vi "OpenSF.vi"(1 "Port number\nactuators":u16, 2 "Port number\nsensors":u16) -> (0 "connection IDs":T1)   [LabVIEW 2010]
panel:
  out "Error out\nactuators":errorcluster
  out "Error out\nsensors":errorcluster
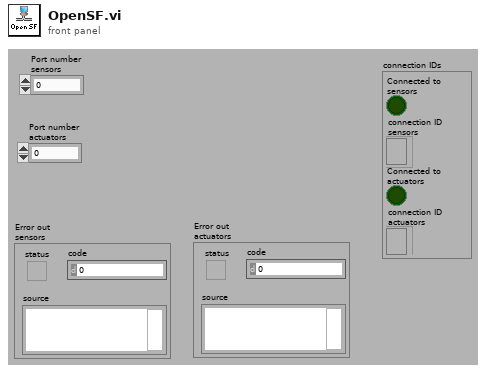
[diagram p1: front panel]
types:
  T1 = cluster{"Connected to\nsensors":bool, "connection ID\nsensors":refnum<k5>, "Connected to\nactuators":bool, "connection ID\nactuators":refnum<k5>}
  T2 = cluster{bool, "connection ID":refnum<k5>, bool, "connection ID":refnum<k5>}
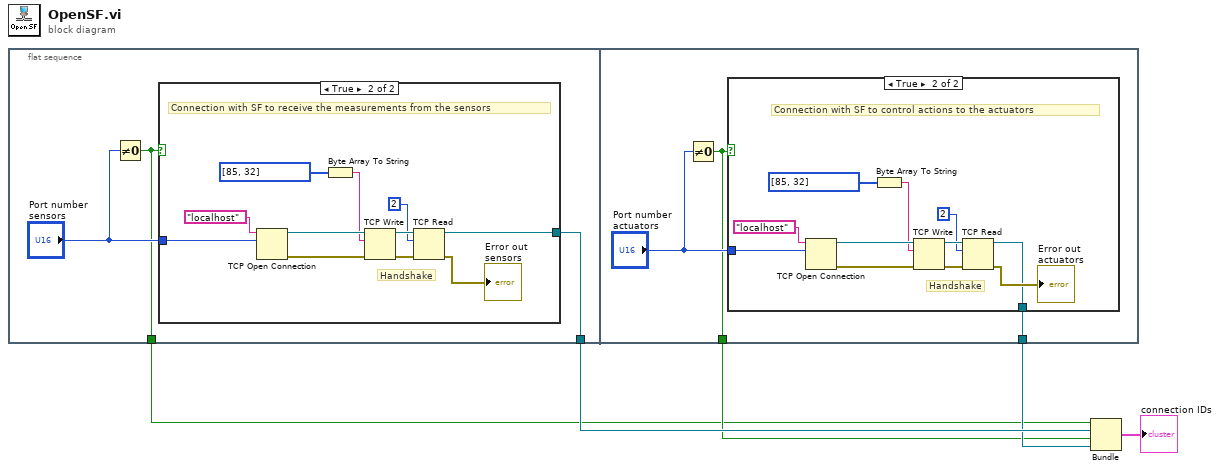
[diagram p0: block diagram]
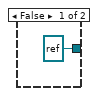
[diagram p2: hidden frame]
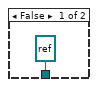
[diagram p3: hidden frame]
diagram:
  n1 = flat-sequence {
    tunnel: [w8] -> w5
    tunnel: [w6] -> w1
    tunnel: [w23] -> w4
    tunnel: [w21] -> w2
    frame #0 {
      n2 = Not Equal To 0?(x="Port number\nsensors") -> (x != 0?=w6:bool)
      n3 = case shown="True" w6 {
        tunnel: "Port number\nsensors" -> [_ w19]
        tunnel: [refnum<k5> refnum ("connection ID") w10] -> w8
        frame False {
        }
        frame True {
          # "Connection with SF to receive the measurements from the sensors"
          # "Handshake"
          n4 = TCP Open Connection(address="localhost", remote port or service name=w19) -> (connection ID=w16:refnum<k5>, error out=w15:errorcluster)  [unwired: 3 in]
          n5 = Byte Array To String(unsigned byte array=u8[] [85, 32]) -> (string=w12:string)
          n6 = TCP Write(connection ID=w16, data in=w12, error in (no error)=w15) -> (connection ID out=w17:refnum<k5>, error out=w18:errorcluster)  [unwired: 1 in, 1 out]
          n7 = TCP Read(connection ID=w17, bytes to read=2, error in (no error)=w18) -> (connection ID out=w10:refnum<k5>, error out=→"Error out\nsensors":errorcluster)  [unwired: 2 in, 1 out]
        }
      }
    }
    frame #1 {
      n8 = Not Equal To 0?(x="Port number\nactuators") -> (x != 0?=w21:bool)
      n9 = case shown="True" w21 {
        tunnel: "Port number\nactuators" -> [_ w34]
        tunnel: [refnum<k5> refnum ("connection ID") w25] -> w23
        frame False {
        }
        frame True {
          # "Connection with SF to control actions to the actuators"
          # "Handshake"
          n10 = TCP Open Connection(address="localhost", remote port or service name=w34) -> (connection ID=w31:refnum<k5>, error out=w30:errorcluster)  [unwired: 3 in]
          n11 = Byte Array To String(unsigned byte array=u8[] [85, 32]) -> (string=w27:string)
          n12 = TCP Write(connection ID=w31, data in=w27, error in (no error)=w30) -> (connection ID out=w32:refnum<k5>, error out=w33:errorcluster)  [unwired: 1 in, 1 out]
          n13 = TCP Read(connection ID=w32, bytes to read=2, error in (no error)=w33) -> (connection ID out=w25:refnum<k5>, error out=→"Error out\nactuators":errorcluster)  [unwired: 2 in, 1 out]
        }
      }
    }
  }
  n14 = Bundle(w1, "connection ID"=w5, w2, "connection ID"=w4) -> (→"connection IDs":T2)  [unwired: 1 in]
